vi "read_attributes.vi"(8 "error in (no error)":errorcluster, 11 "MLPClassifier in":refnum<class "MLPClassifier.lvclass">) -> (0 "error out":errorcluster, 2 "attributes":T1, 3 "MLPClassifier out":refnum<class "MLPClassifier.lvclass">)   [LabVIEW 2020, in "MLPClassifier.lvclass"]
uses:
  MLPClassifier.lvclass
  Controls/mlp_classifier_attributes.ctl
  MLPClassifier.lvclass/MLPClassifier.ctl
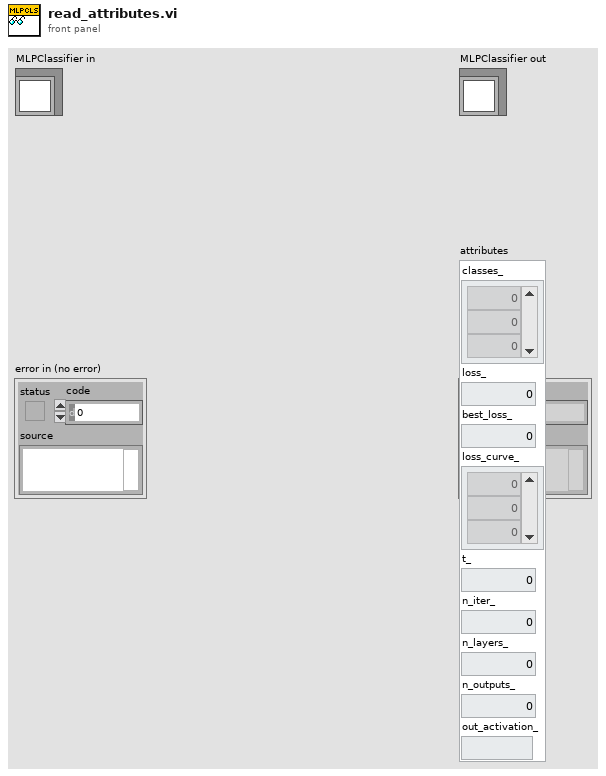
[diagram p1: front panel]
types:
  T1 = typedef "mlp_classifier_attributes.ctl" = cluster{"classes_":dbl[][], "loss_":dbl, "best_loss_":dbl, "loss_curve_":dbl[], "t_":dbl, "n_iter_":dbl, "n_layers_":dbl, "n_outputs_":dbl, "out_activation_":string}
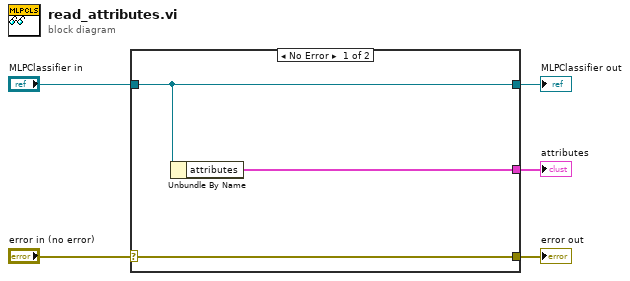
[diagram p0: block diagram]
diagram:
  n1 = case shown="No Error" "error in (no error)" {
    selector: "error in (no error)" -> [w8 w9]
    tunnel: [w8 w9] -> w4
    tunnel: [w7 w10] -> w2
    tunnel: "MLPClassifier in" -> [w7 w10]
    tunnel: [w6 _] -> w1
    frame No Error {
      n2 = Unbundle By Name(w7) -> ("attributes"=w6:T1)
    }
    frame Error {
    }
  }
  "error out" <- w4
  "MLPClassifier out" <- w2
  "attributes" <- w1
